vi "BUILD_vipb path.vi"() -> (2 "2":path, 3 "appended path":path)   [LabVIEW 2013]
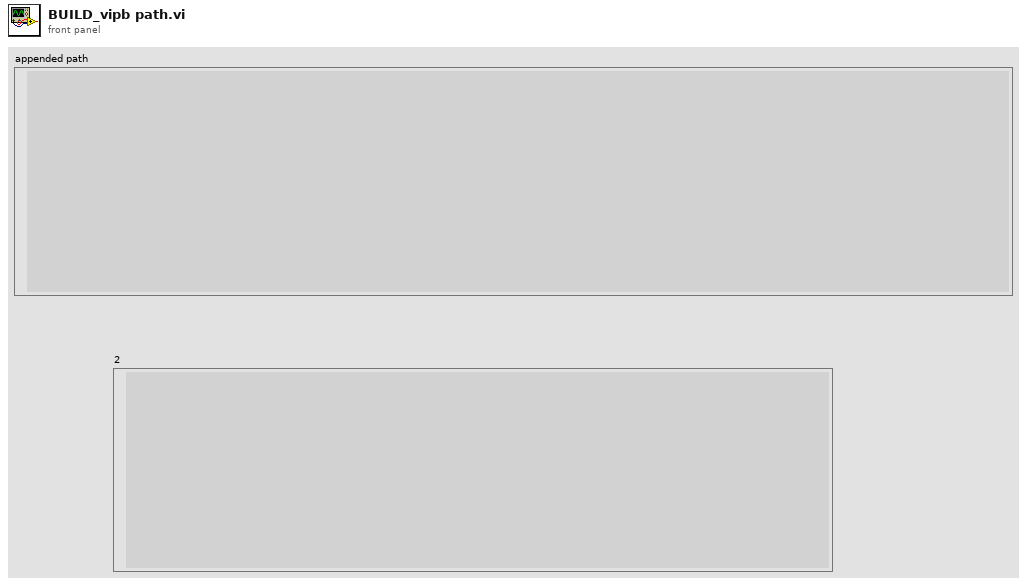
[diagram p1: front panel]
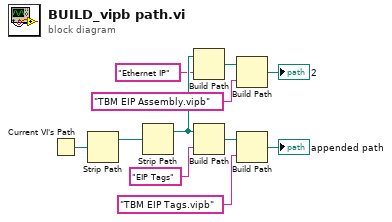
[diagram p0: block diagram]
diagram:
  n1 = Current VI's Path() -> (path=w9:path)
  n2 = Strip Path(path=w9) -> (stripped path=w10:path)  [unwired: 1 out]
  n3 = Strip Path(path=w10) -> (stripped path=w7:path)  [unwired: 1 out]
  n4 = Build Path(base path=w7, name or relative path="Ethernet IP") -> (appended path=w5:path)
  n5 = Build Path(base path=w7, name or relative path="EIP Tags") -> (appended path=w4:path)
  n6 = Build Path(base path=w5, name or relative path="TBM EIP Assembly.vipb") -> (appended path=→"2":path)
  n7 = Build Path(base path=w4, name or relative path="TBM EIP Tags.vipb") -> (appended path=→"appended path":path)
